vi "Write Msg Header.vi"(7 "Sender Name":string, 8 "error in (no error)":errorcluster, 9 "Time Stamp":timestamp, 10 "Msg ID":T1, 11 "RDS Message in":refnum<class "RDS Message.lvclass">) -> (0 "error out":errorcluster, 3 "RDS Message out":refnum<class "RDS Message.lvclass">)   [LabVIEW 2015, in "RDS Child Messages.lvlib" / "RDS Message.lvclass"]
uses:
  RDS Message.lvclass
  RDS Message ID.ctl
  RDS Message.lvclass/RDS Message.ctl
  RDS Child Messages/RDS Child Messages.lvlib
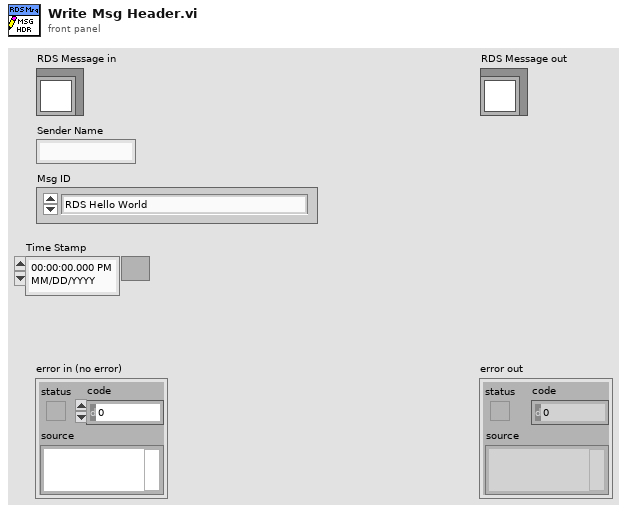
[diagram p1: front panel]
types:
  T1 = typedef "RDS Child Messages.lvlib/RDS Message ID.ctl" = enum16{"RDS Hello World", "String Message", "AIP_Status", "AIP_Command", "GPS_Data", "MCB_Command", "MCB_Status", "Compass_Data", "Depth_Data", "Battery_Data", "Contoller_State", "Set_Mag_Dev", "BTB_Shutdown", "State_Sample_Request", "State_Sample", "PID_Gains_Set", "Helm_Limiter_Set", "Helm_Heading_Command", "Helm_Steering_Command", "Helm_Status", "Controller_Message", "AIP_Set_Min_Depth", "Mission_Controller_State", "Mission_Upload", "Mission_Set_Op_and_Run", "Mission_Settings_Set"}
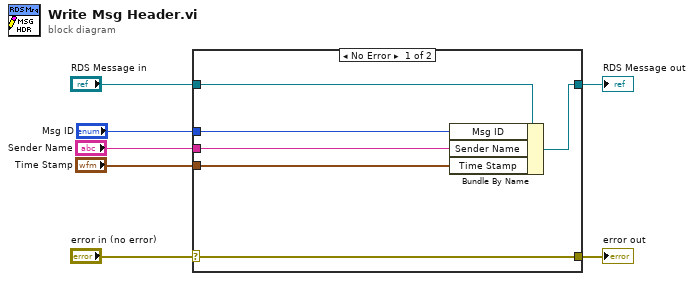
[diagram p0: block diagram]
diagram:
  n1 = case shown="No Error" "error in (no error)" {
    selector: "error in (no error)" -> [w13 w14]
    tunnel: [w13 w14] -> w6
    tunnel: [w11 w15] -> w4
    tunnel: "RDS Message in" -> [w12 w15]
    tunnel: "Sender Name" -> [w10 _]
    tunnel: "Time Stamp" -> [w9 _]
    tunnel: "Msg ID" -> [w8 _]
    frame No Error {
      n2 = Bundle By Name(cluster=w12, "Msg ID"=w8, "Sender Name"=w10, "Time Stamp"=w9) -> (w11:refnum<class "RDS Message.lvclass">)
    }
    frame Error {
    }
  }
  "error out" <- w6
  "RDS Message out" <- w4
